vi "ToRepo.vi"(8 "error in":errorcluster, 9 "to repo cluster":T1, 10 "repository in":refnum<class "NISE_CEF_Repository.lvclass">, 11 "group in":refnum<class "device.lvclass">) -> (0 "error out":errorcluster, 2 "repository out":refnum<class "NISE_CEF_Repository.lvclass">, 3 "group out":refnum<class "device.lvclass">)   [LabVIEW 2013, in "device.lvclass"]
uses:
  device.lvclass
  <vilib>/NI/Configuration Framework/Repository/NISE_CEF_Repository.lvclass
  <vilib>/NI/Configuration Framework/Node/ToRepoCluster.ctl
  <vilib>/NI/Configuration Framework/Node/NISE_CEF_Node.lvclass
  device.lvclass/device.ctl
  database file/database file.lvclass
  database file/database file.lvclass/database file.ctl
  database file/Write frames.vi
  database file/Read frames.vi
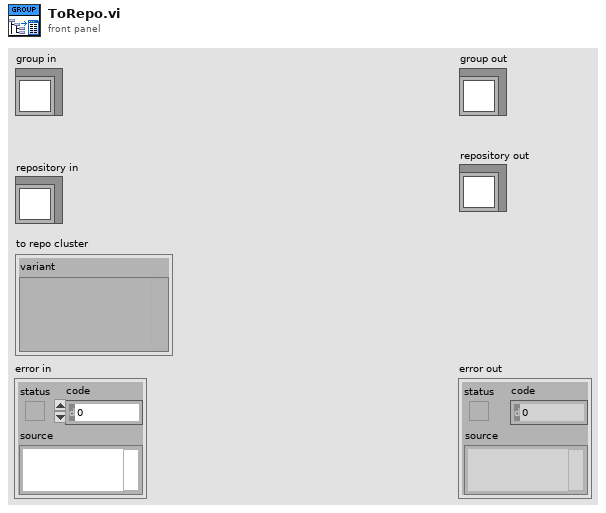
[diagram p1: front panel]
types:
  T1 = typedef "NISE_CEF_Node.lvclass/ToRepoCluster.ctl" = cluster{"variant":variant}
  T2 = typedef "J1939.lvlib/J1939 db frame.ctl" = cluster{"name":string, "Priority":u8, "PGN":u32, "Reserved Bit":u8, "Data page":u8, "PDU Format":u8, "PDU Specific":u8, "Source Address":u8, "PayldLen":u32, "signals":T3[], "Comment":string, "can timing type":u32, "transmit time":dbl, "direction":u16}
  T3 = typedef "J1939.lvlib/J1939 db signal.ctl" = cluster{"NameShort":string, "SPN":i32, "StartBit":u32, "NumBits":u32, "DataType":u32, "ByteOrdr":u32, "ScaleFac":dbl, "ScaleOff":dbl, "Max":dbl, "Min":dbl, "Default":dbl, "Unit":string, "Comment":string}
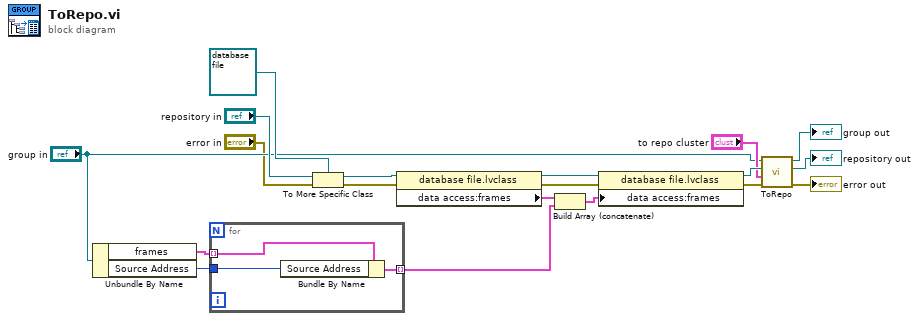
[diagram p0: block diagram]
diagram:
  n1 = Unbundle By Name("group in") -> ("frames"=w5:T2[], "Source Address"=w4:u8)
  n2 = for {
    tunnel: w5 -> [w22] mode=indexing
    tunnel: w4 -> [w21]
    tunnel: [w20] -> w3 mode=indexing
    n3 = Bundle By Name(cluster=w22, "Source Address"=w21) -> (w20:T2)
  }
  n4 = To More Specific Class(target class=refnum<class "database file.lvclass"> refnum ("cRIO repo.lvclass"), reference="repository in", error in="error in") -> (specific class reference=w10:refnum<class "database file.lvclass">, error out=w1:errorcluster)
  n5 = property class="database file.lvclass"(reference=w10, error in=w1) -> (reference out=w9:refnum<class "database file.lvclass">, error out=w11:errorcluster, "data access:frames"=w8:T2[])
  n6 = Build Array (concatenate)(w8, w3) -> (w7:T2[])
  n7 = property class="database file.lvclass"(reference=w9, error in=w11, "data access:frames"=w7) -> (reference out=w14:refnum<class "database file.lvclass">, error out=w13:errorcluster)
  n8 = call-parent "ToRepo.vi"("error in"=w13, "to repo cluster"="to repo cluster", "repository in"=w14, "node in"="group in") -> ("error out"=→"error out":errorcluster, "repository out"=→"repository out":refnum<class "NISE_CEF_Repository.lvclass">, "node out"=→"group out":refnum<class "device.lvclass">)  [unwired: 5 in]
